vi "SPMain.vi"   [LabVIEW 2014]
uses:
  <vilib>/Platform/TimedLoop/XDataNode/timing_clust.ctl
  <vilib>/Platform/TimedLoop/XDataNode/nitl_modes.ctl
  <vilib>/Platform/TimedLoop/XDataNode/wakeup.ctl
  <vilib>/rvi/Emulation/niFpgaSctlEmulationGetInTimedLoop.vi
  <vilib>/rvi/Emulation/niFpgaEmulationReportErrorSimple.vi
  <vilib>/rvi/Emulation/niFpgaGetClockAttributes.vi
  <vilib>/rvi/Emulation/niFpgaCriticalErrorInLSC.vi
  <vilib>/rvi/Emulation/niFpgaProcessEmulError.vi
  <vilib>/rvi/eio/common/nirviEmuTemplateMethod_errors.vi
  simpleCounterGlobals.vi
  <vilib>/Platform/TimedLoop/XDataNode/XDataNode.xnode
  <vilib>/eio/EIONode/EIONode.xnode
  <vilib>/Platform/TimedLoop/XDataNode/XDNodeRunTimeDep.lvlib
types:
  T1 = typedef "XDNodeRunTimeDep.lvlib/timing_clust.ctl" = cluster{"Expected End [f-1]":u64, "Actual End [f-1]":u64, "Finished Late? [f-1]":bool, "Expected End [i-1]":u64, "Actual End [i-1]":u64, "Finished Late? [i-1]":bool, "Expected Start [i]":u64, "Actual Start [i]":u64, "Expected Start [f]":u64, "Actual Start [f]":u64, "Source Name":string, "Structure Name":string, "Period":i64, "Deadline":i64, "Offset":i64, "Start":i64, "Priority":i32, "Timeout":i32, "Mode":T2, "Wakeup Reason":T3, "Error":errorcluster, "Source Type":string, "Secondary Source Type":string, "Global End Time":u64, "Global Start Time":u64, "Frame Duration":u64, "Iteration Duration":u64, "Assigned CPU":i32, "I/O Scan Engine Mode":u32}
  T2 = typedef "XDNodeRunTimeDep.lvlib/nitl_modes.ctl" = enum32{"No Change", "Process missed periods, maintain original phase", "Discard missed periods, maintain original phase", "Process missed periods, ignore original phase", "Discard missed periods, ignore original phase"}
  T3 = typedef "XDNodeRunTimeDep.lvlib/wakeup.ctl" = enum32{"Normal", "Aborted", "Asynchronous wakeup", "Timing source error", "Timed loop error", "Timeout"}
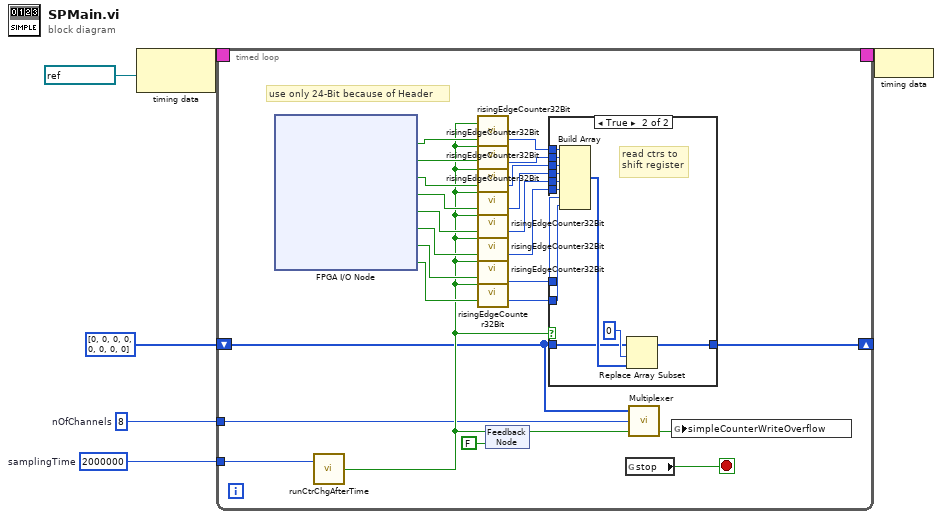
[diagram p0: block diagram]
diagram:
  w1 = u32 2000000  # samplingTime
  w2 = u8 8  # nOfChannels
  n1 = node-c288(refnum<k21> "100MHz" ("Source Name")) -> (w6:T1)
  n2 = timed-loop {
    timing: w6 -> [_]
    timing-out: [_] -> w5
    shift-right: [w15] -> _
    shift-left: u32[] [0, 0, 0, 0, 0, 0, 0, 0] -> [w11]
    tunnel: w2 -> [w9]
    tunnel: w1 -> [w14]
    stop <- w8 stop-if-true
    # "use only 24-Bit because of Header"
    n3 = xnode "FPGA I/O Node"() -> ("Connector1/DIO32"=w31:bool, "Connector1/DIO33"=w30:bool, "Connector1/DIO34"=w29:bool, "Connector1/DIO35"=w28:bool, "Connector1/DIO36"=w27:bool, "Connector1/DIO37"=w26:bool, "Connector1/DIO38"=w25:bool, "Connector1/DIO39"=w24:bool)  [unwired: 8 in, 8 out]
    n4 = call "runCtrChgAfterTime.vi"("timeDif(ticks)"=w14) -> ("change"=w13:bool)  [unwired: 1 in]
    n5 = call "risingEdgeCounter32Bit.vi"("In"=w31, "Reset"=w13) -> ("32BitCounter"=w23:u32)  [unwired: 1 in]
    n6 = call "risingEdgeCounter32Bit.vi"("In"=w30, "Reset"=w13) -> ("32BitCounter"=w22:u32)  [unwired: 1 in]
    n7 = call "risingEdgeCounter32Bit.vi"("In"=w29, "Reset"=w13) -> ("32BitCounter"=w21:u32)  [unwired: 1 in]
    n8 = call "risingEdgeCounter32Bit.vi"("In"=w28, "Reset"=w13) -> ("32BitCounter"=w20:u32)  [unwired: 1 in]
    n9 = call "risingEdgeCounter32Bit.vi"("In"=w27, "Reset"=w13) -> ("32BitCounter"=w19:u32)  [unwired: 1 in]
    n10 = call "risingEdgeCounter32Bit.vi"("In"=w26, "Reset"=w13) -> ("32BitCounter"=w18:u32)  [unwired: 1 in]
    n11 = call "risingEdgeCounter32Bit.vi"("In"=w25, "Reset"=w13) -> ("32BitCounter"=w17:u32)  [unwired: 1 in]
    n12 = call "risingEdgeCounter32Bit.vi"("In"=w24, "Reset"=w13) -> ("32BitCounter"=w16:u32)  [unwired: 1 in]
    n13 = feedback-in #1(w13) -> ()
    n14 = feedback #1(FALSE ("change")) -> (w10:bool)
    n15 = case shown="True" w13 {
      tunnel: w23 -> [_ w44]
      tunnel: w22 -> [_ w43]
      tunnel: w21 -> [_ w42]
      tunnel: w20 -> [_ w41]
      tunnel: w19 -> [_ w40]
      tunnel: w18 -> [_ w39]
      tunnel: w17 -> [_ w38]
      tunnel: w16 -> [_ w37]
      tunnel: [w32 w34] -> w15
      tunnel: w11 -> [w32 w33]
      frame False {
      }
      frame True {
        # "read ctrs to\nshift register"
        n16 = Build Array(w44, w43, w42, w41, w40, w39, w38, w37) -> (w36:u32[])
        n17 = Replace Array Subset(array=w33, new element=w36, index=0) -> (w34:u32[])
      }
    }
    n18 = global read "simpleCounterGlobals.vi" "stop"() -> (w8:bool)
    n19 = call "Multiplexer.vi"("write"=w10, "nOfChannels"=w9, "Data"=w11) -> ("Timed Out?"=w7:bool)  [unwired: 2 in]
    n20 = global write "simpleCounterGlobals.vi" "simpleCounterWriteOverflow"(w7) -> ()
  }
  n21 = node-c288(w5) -> ()
